vi "State_Machine.vi"(8 "error in (no error)":errorcluster caption="entrée d'erreur (pas d'erreur)", 11 "Get_Voltage en entrée":refnum<class "Pattern_Matching.lvclass">) -> (0 "error out":errorcluster caption="sortie d'erreur", 2 "Json_String":string, 3 "Get_Voltage en sortie":refnum<class "Pattern_Matching.lvclass">)   [LabVIEW 2020, in "Library Test.lvlib" / "Pattern_Matching.lvclass"]
uses:
  Pattern_Matching.lvclass
  C:/Users/ngarcin/OneDrive - Altyor/Standard TB/Class/Test/Test (Default)/Test (Default).lvclass
  JSON API/JSON Value/Set from JSON string.vi
  Instrument/Instrument (Default)/Class Instrument (Default).lvclass
  JSON API/JSON Value/JSON Value.lvclass
  Pattern_Matching.lvclass/Pattern_Matching.ctl
  JSON API/Variant JSON/Variant JSON.lvlib
  JSON API/Get Polymorphic/JSON GetSet.lvlib
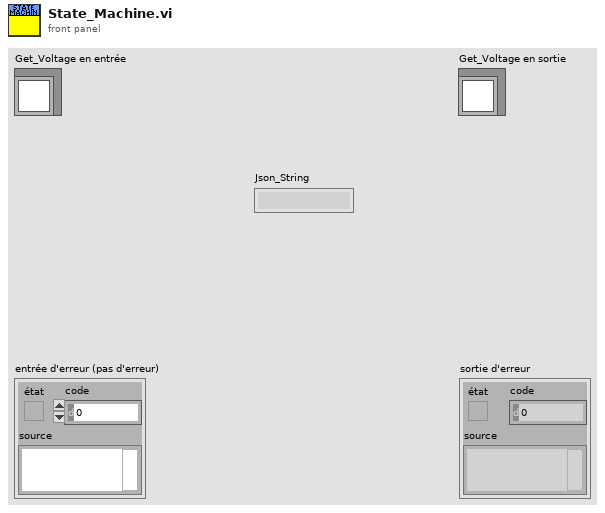
[diagram p1: front panel]
types:
  T1 = cluster{"Result Test":bool, "Result Value":string}
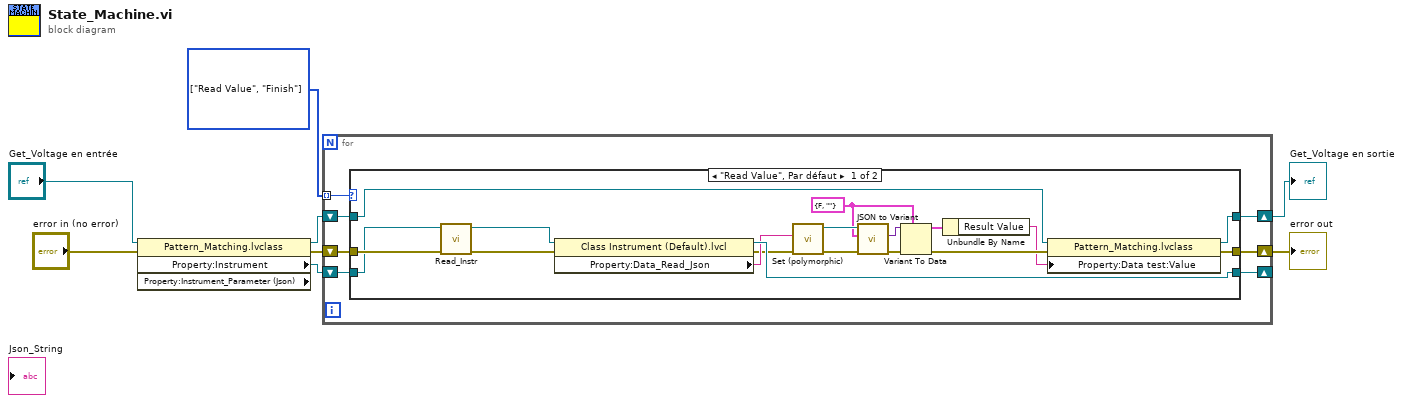
[diagram p0: block diagram]
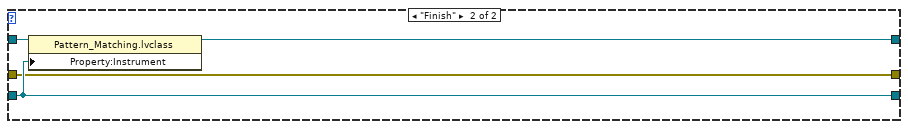
[diagram p2: hidden frame]
diagram:
  w7 = enum16{"Init", "Read Value", "Finish"}[] [enum."Read Value", enum."Finish"] items=["Init", "Read Value", "Finish"]
  n1 = property class="Pattern_Matching.lvclass" props=["Property:Instrument", "Property:Instrument_Parameter (Json)"](reference="Get_Voltage en entrée", error in="error in (no error)") -> (reference out=w5:refnum<class "Pattern_Matching.lvclass">, error out=w1:errorcluster, "Property:Instrument"=w6:refnum<class "Class Instrument (Default).lvclass">)  [unwired: 1 out]
  n2 = for {
    tunnel: w7 -> [w15] mode=indexing
    shift-right: [w13] -> _
    shift-left: w6 -> [w14]
    shift-right: [w11] -> w3
    shift-left: w5 -> [w12]
    shift-right: [w9] -> w4
    shift-left: w1 -> [w10]
    n3 = case shown="\"Read Value\", Par défaut" w15 {
      tunnel: w14 -> [w16 w35]
      tunnel: [w31 w35] -> w13
      tunnel: w12 -> [w33 w37]
      tunnel: [w21 w36] -> w11
      tunnel: w10 -> [w17 w34]
      tunnel: [w30 w34] -> w9
      frame "Read Value", Default {
        w20 = T1 {"Result Test"=FALSE, "Result Value"=""}
        n4 = call-dynamic "Read_Instr.vi"("error in (no error)"=w17, "Class Instrument (Default) en entrée"=w16) -> ("error out"=w29:errorcluster, "Class Instrument (Default) en sortie"=w32:refnum<class "Class Instrument (Default).lvclass">)  [unwired: 8 in]
        n5 = property class="Class Instrument (Default).lvcl"(reference=w32, error in=w29) -> (reference out=w31:refnum<class "Class Instrument (Default).lvclass">, error out=w24:errorcluster, "Property:Data_Read_Json"=w25:string)
        n6 = call-poly "Set (polymorphic).vi"("error in (no error)"=w24, "JSON stream"=w25) -> ("error out"=w28:errorcluster, "JSON Value out"=w26:refnum<class "JSON Value.lvclass">)  [unwired: 7 in, 1 out]
        n7 = call "JSON to Variant.vi"("error in (no error)"=w28, "Variant (Data Type)"=w20, "JSON Value"=w26) -> ("error out"=w27:errorcluster, "Variant out"=w23:variant)  [unwired: 7 in]
        n8 = Variant To Data(error in=w27, type=w20, Variant=w23) -> (data=w19:T1, error out=w22:errorcluster)
        n9 = Unbundle By Name(w19) -> ("Result Value"=w18:string)
        n10 = property class="Pattern_Matching.lvclass"(reference=w33, error in=w22, "Property:Data test:Value"=w18) -> (reference out=w21:refnum<class "Pattern_Matching.lvclass">, error out=w30:errorcluster)
      }
      frame "Finish" {
        n11 = property class="Pattern_Matching.lvclass"(reference=w37, "Property:Instrument"=w35) -> (reference out=w36:refnum<class "Pattern_Matching.lvclass">)  [unwired: 1 in, 1 out]
      }
    }
  }
  "error out" <- w4
  "Get_Voltage en sortie" <- w3
